vi "AO_master_Widefield_v0.vi"() -> ()   [LabVIEW 2018]
panel:
  in  "TurnOFFCooler":bool=TRUE caption="PD Correction"
  out "Return from GetStatus":u32
  in  "488 shutter":refnum<k7>(container)
  in  "Current Z as Center":bool=TRUE caption="PD Correction"
  in  "Z Step Num":i32=7
  in  "Z Step Size (um)":dbl=0.2
  in  "Spool":bool=TRUE caption="Cameras Live Display"
  in  "Acquire":bool
  in  "VISA Stage":refnum<visa-resource-name>="COM5"
  in  "Stage Options":bool
  in  "Auto Scale":bool=TRUE caption="PD Correction"
  out "Get EMCCD Gain":i32=1
  out "Return from SetSpool":i32=1
  out "Running Status":T1(ring) caption="Camera FOV"
  out "Return from Start Acquisition":u32
  out "Return from GetAcquiredData":u32
  in  "Folder Name":string="test"
  in  "File Type":enum16{"TIFF", "Sif"}(ring)
  out "Return from CheckProcess":u32
  out "Get Kinetic Time":sgl format="%.4f"
  out "Get Accum Time":sgl format="%.4f"
  out "Get Kinetic Num":i32=1
  out "Get Accum Num":i32=1
  in  "Abort":bool
  out "FOV Y Pixels":i32
  out "FOV X Pixels":i32
  in  "Snap":bool
  in  "Exit":bool
  out "EMCCD Status":bool
  in  "Stop LIVE":bool
  in  "Start LIVE":bool
  out "error out":errorcluster
  out "Return from CheckTimings":u32
  out "Get Exposure Time":sgl format="%.4f"
  in  "error in (no error)":errorcluster
  in  "Intensity Min":dbl=200.0 min=1.0
  in  "Intensity Max":dbl=10000.0 min=1.0
  in  "Shutdown EMCCD when exit":bool=TRUE caption="PD Correction"
  in  "Update FOV":bool
  in  "Update AcqSetting":bool
  in  "Exposure time (s)":dbl=0.02
  in  "Main Path":path=path "D:/Data"
  in  "File Name":string="test"
  in  "Kinetic Num":u32=1
  in  "Accum Num":u32=1
  in  "Initialize EMCCD":bool=TRUE caption="PD Correction"
  in  "CoolToTargetTemp":bool=TRUE caption="PD Correction"
  out "Intensity Graph":i32[][](graph)
  out "Current Temp":i32
  out "Detector Y Pixels":i32
  out "Detector X Pixels":i32
  in  "Aquisition Mode":T2(ring)=enum."Single Scan" caption="Camera FOV"
  in  "Trigger Mode":enum16{"Internal", "External"}(ring) caption="Camera FOV"
  in  "Gain Value":sgl=20.0 format="%.2f"
  in  "Yend":i32=1002
  in  "Xend":i32=1004
  in  "Ystart":i32=2
  in  "Xstart":i32=2
  in  "Ybin":i32=1
  in  "Xbin":i32=1
  in  "Camera FOV":T3(ring)=enum."Full FOV"
  in  "Gain On":bool=TRUE caption="Cameras Live Display"
  in  "Set Temp":i32=-60
  # "To do:\n1. make Kinetic work\n2. Gain setting\n3. live stage operation"
  # "It takes some time to cool down the camera before it shutdowns"
  # "C"
  # "Z move by relative position"
  # "Acquisition Settings"
  # "Status"
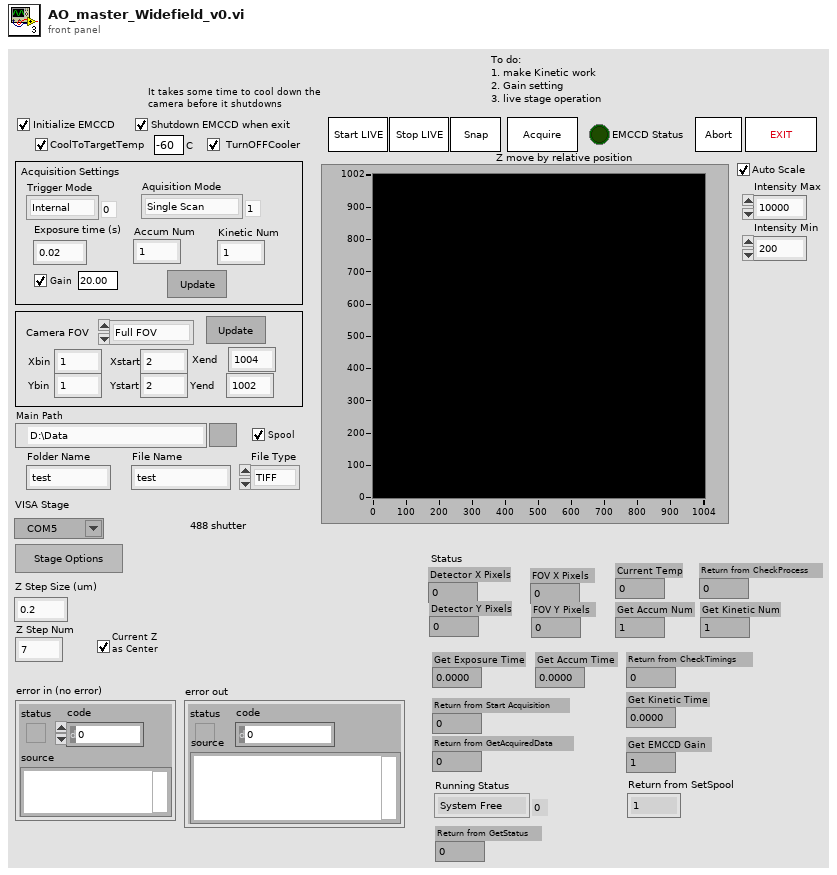
[diagram p1: front panel]
types:
  T1 = enum16{"System Free", "Live Preview", "Snap", " Acquisition", ""}
  T2 = enum16{"None", "Single Scan", "Accumulate", "Kinetics", "Fast Kinetics", "Run till abort"}
  T3 = enum16{"Custom FOV", "Full FOV", "FOV: 768x768", "FOV: 512x512", "FOV: 320x320", "FOV: 256x256", ""}
  T4 = typedef "Error Code Enum typedef.ctl" = enum32{"N/A (0)", "DRV_ERROR_CODES", "DRV_SUCCESS", "DRV_VXDNOTINSTALLED", "DRV_ERROR_SCAN", "DRV_ERROR_CHECK_SUM", "DRV_ERROR_FILELOAD", "DRV_UNKNOWN_FUNC", "DRV_ERROR_VXD_INIT", "DRV_ERROR_ADDRESS", "DRV_ERROR_PAGELOCK", "DRV_ERROR_PAGEUNLOCK", "DRV_ERROR_BOARDTEST", "DRV_ERROR_ACK", "DRV_ERROR_UP_FIFO", "DRV_ERROR_PATTERN", "N/A (16)", "DRV_ACQUISITION_ERRORS", "DRV_ACQ_BUFFER", "DRV_ACQ_DOWNFIFO_FULL", "DRV_PROC_UNKONWN_INSTRUCTION", "DRV_ILLEGAL_OP_CODE", "DRV_KINETIC_TIME_NOT_MET", "DRV_ACCUM_TIME_NOT_MET", "DRV_NO_NEW_DATA", "N/A (25)", "DRV_SPOOLERROR", "N/A (27)", "N/A (28)", "N/A (29)", "N/A (30)", "N/A (31)", "N/A (32)", "DRV_TEMPERATURE_CODES", "DRV_TEMPERATURE_OFF", "DRV_TEMPERATURE_NOT_STABILIZED", "DRV_TEMPERATURE_STABILIZED", "DRV_TEMPERATURE_NOT_REACHED", "DRV_TEMPERATURE_OUT_RANGE", "DRV_TEMPERATURE_NOT_SUPPORTED", "DRV_TEMPERATURE_DRIFT", "N/A (41)", "N/A (42)", "N/A (43)", "N/A (44)", "N/A (45)", "N/A (46)", "N/A (47)", "N/A (48)", "DRV_GENERAL_ERRORS", "DRV_INVALID_AUX", "DRV_COF_NOTLOADED", "DRV_FPGAPROG", "DRV_FLEXERROR", "DRV_GPIBERROR", "N/A (55)", "N/A (56)", "N/A (57)", "N/A (58)", "N/A (59)", "N/A (60)", "N/A (61)", "N/A (62)", "N/A (63)", "DRV_DATATYPE", "DRV_DRIVER_ERRORS", "DRV_P1INVALID", "DRV_P2INVALID", "DRV_P3INVALID", "DRV_P4INVALID", "DRV_INIERROR", "DRV_COFERROR", "DRV_ACQUIRING", "DRV_IDLE", "DRV_TEMPCYCLE", "DRV_NOT_INITIALIZED", "DRV_P5INVALID", "DRV_P6INVALID", "DRV_INVALID_MODE", "DRV_INVALID_FILTER", "DRV_I2CERRORS", "DRV_I2CDEVNOTFOUND", "DRV_I2CTIMEOUT", "DRV_P7INVALID", "N/A (84)", "N/A (85)", "N/A (86)", "N/A (87)", "N/A (88)", "N/A (89)", "DRV_IOCERROR", "DRV_VRMVERSIONERROR"}
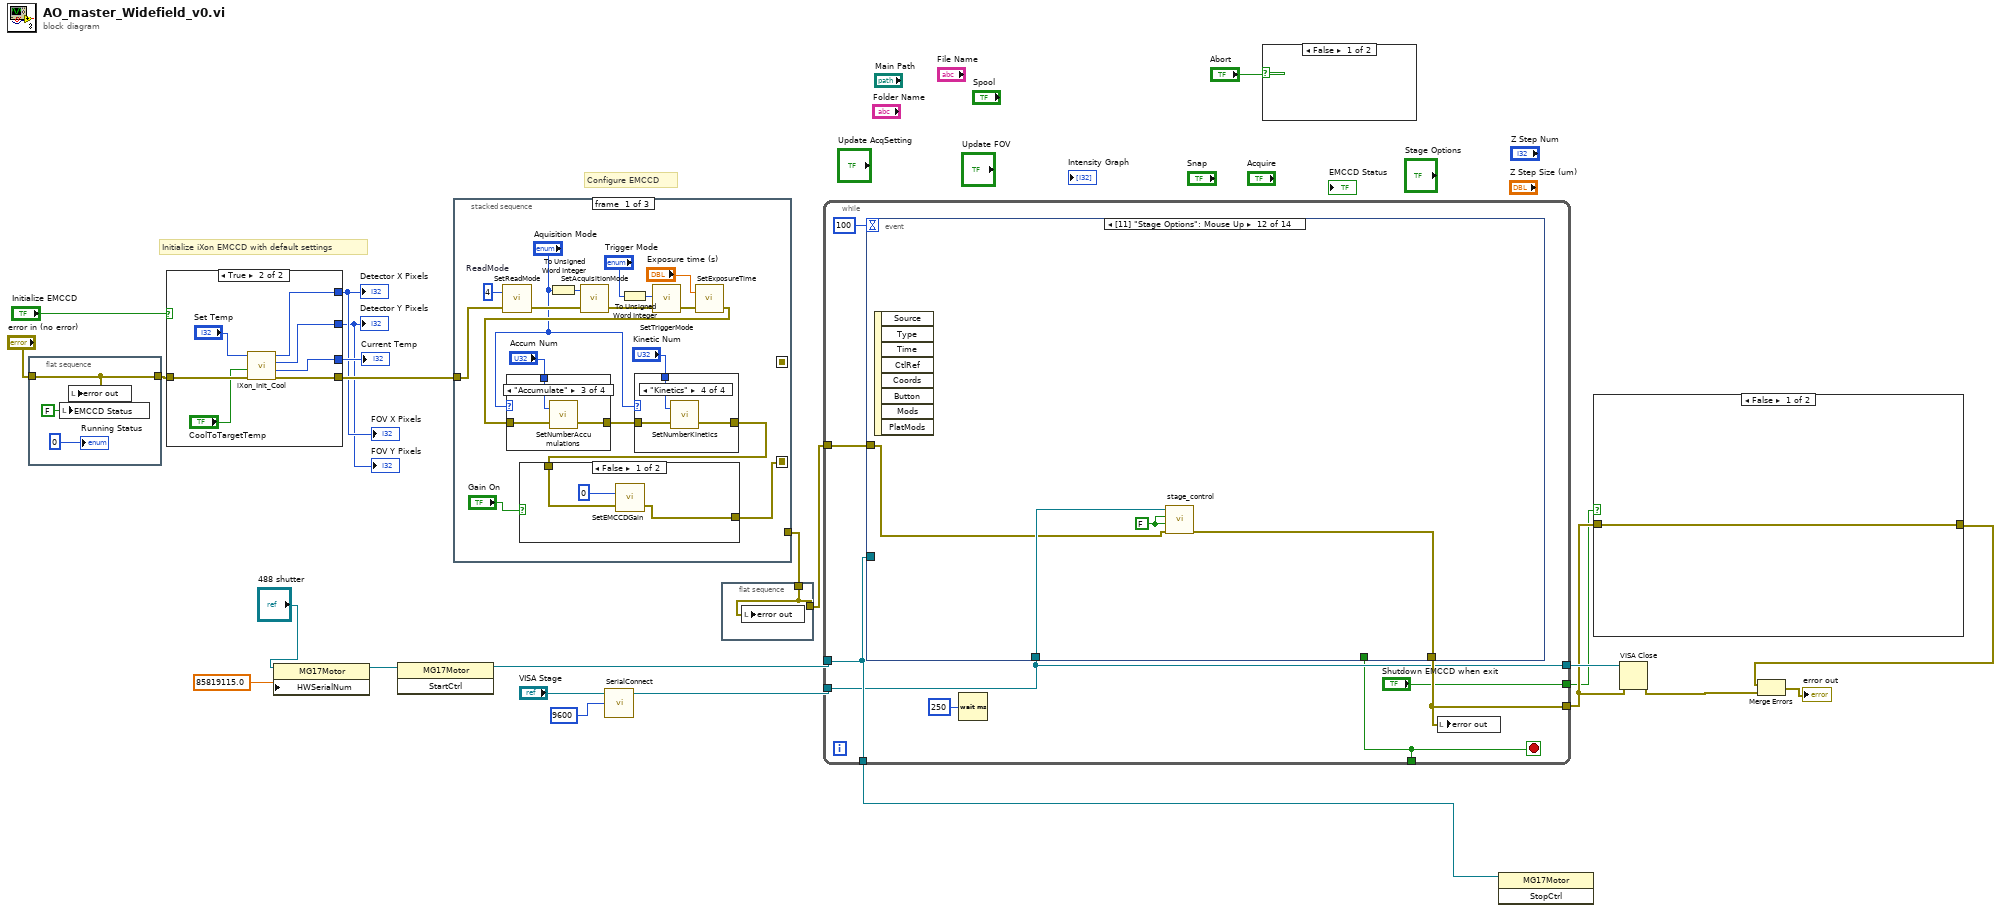
[diagram p0: block diagram]
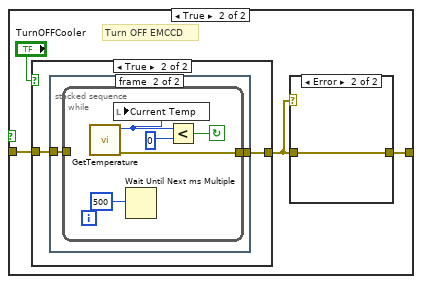
[diagram p2: hidden frame]
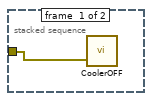
[diagram p4: hidden frame]
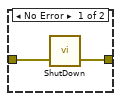
[diagram p5: hidden frame]
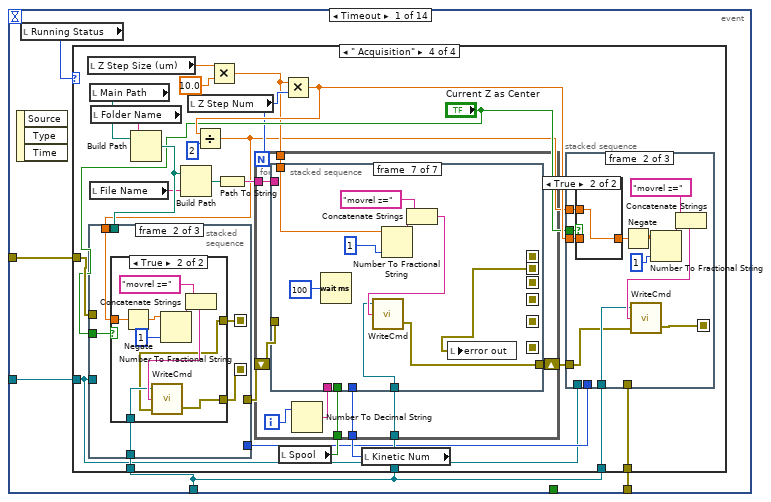
[diagram p7: hidden frame]
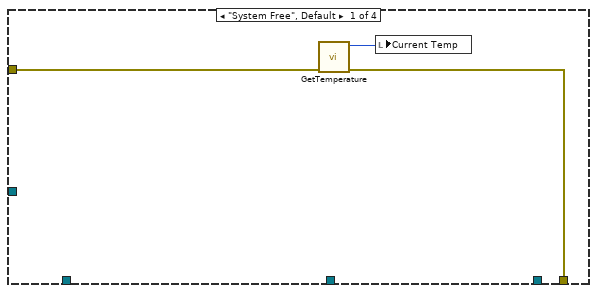
[diagram p8: hidden frame]
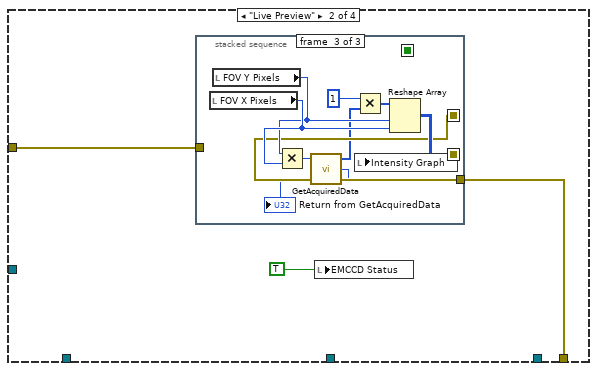
[diagram p9: hidden frame]
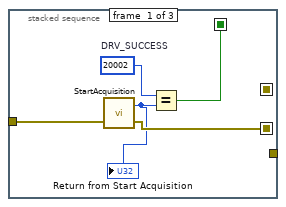
[diagram p10: hidden frame]
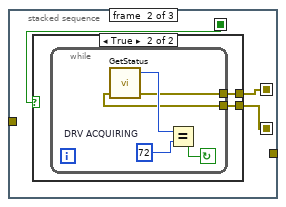
[diagram p11: hidden frame]
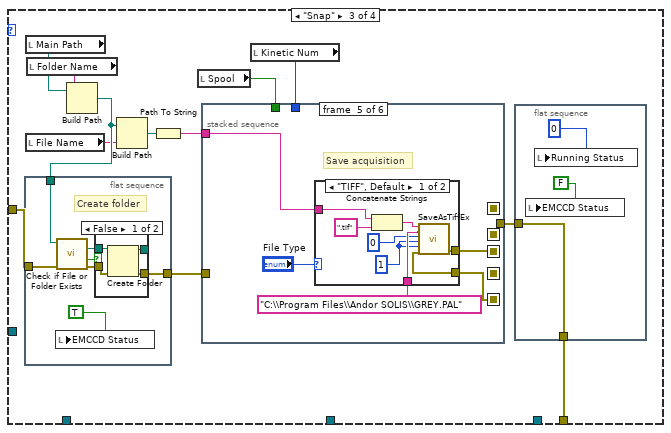
[diagram p13: hidden frame]
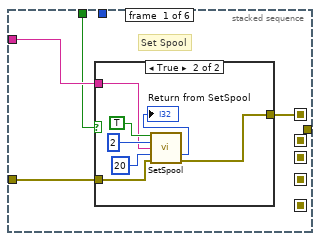
[diagram p14: hidden frame]
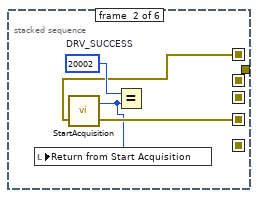
[diagram p16: hidden frame]
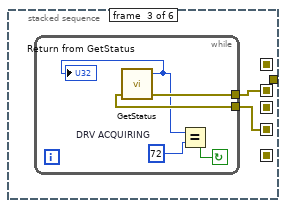
[diagram p17: hidden frame]
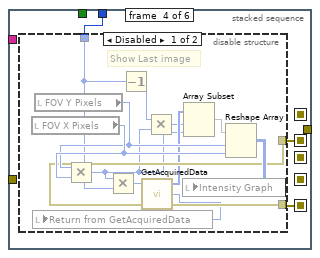
[diagram p18: hidden frame]
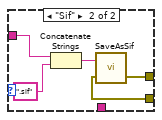
[diagram p20: hidden frame]
diagram:
  # "Configure EMCCD"
  # "Initialize iXon EMCCD with default settings"
  n1 = flat-sequence {
    tunnel: "error in (no error)" -> [w27]
    tunnel: [w27] -> w18
    frame #0 {
      n2 = local write "EMCCD Status"(FALSE) -> ()
      n3 = local write "error out"(w27) -> ()
      "Running Status" <- u16 0
    }
  }
  n4 = case shown="True" "Initialize EMCCD" {
    tunnel: w18 -> [w32 w39]
    tunnel: [w30 w37] -> w21
    tunnel: [w29 w36] -> w20
    tunnel: [w33 w35] -> w23
    tunnel: [w28 w34] -> w22
    frame False {
      n5 = call <userlib>:"GetDetector.vi"("error in (no error)"=w32) -> ("error out"=w31:errorcluster, "ypixels"=w29:i32, "xpixels"=w30:i32)  [unwired: 3 in, 1 out]
      n6 = call <userlib>:"GetTemperature.vi"("error in (no error)"=w31) -> ("error out"=w28:errorcluster, "temperature"=w33:i32)  [unwired: 3 in, 2 out]
    }
    frame True {
      n7 = call "iXon_Init_Cool.vi"("error in (no error)"=w39, "CoolToTargetTemp"="CoolToTargetTemp", "Set Temp"="Set Temp") -> ("error out"=w34:errorcluster, "Current Temp"=w35:i32, "Detector Y Pixels"=w36:i32, "Detector X Pixels"=w37:i32)  [unwired: 5 in]
    }
  }
  "Detector X Pixels" <- w21
  "Detector Y Pixels" <- w20
  "Current Temp" <- w23
  "FOV X Pixels" <- w21
  "FOV Y Pixels" <- w20
  n8 = property class="MG17Motor"(reference="488 shutter", "HWSerialNum"=85819115.0) -> (reference out=w10:refnum<k7>)  [unwired: 1 in, 1 out]
  n9 = invoke class="MG17Motor" method="StartCtrl"(reference=w10) -> (reference out=w7:refnum<k7>)  [unwired: 2 in, 2 out]
  n10 = stacked-sequence {
    seq-local: [w41 _ _] -> [_ w85 _]
    seq-local: [_ w84 _] -> [_ _ w183]
    tunnel: w22 -> [w55 _ _]
    tunnel: [_ _ w175] -> w17
    frame #0 {
      w56 = u16 4  # ReadMode
      n11 = call <userlib>:"SetReadMode.vi"("error in (no error)"=w55, "mode"=w56) -> ("error out"=w53:errorcluster)  [unwired: 1 out]
      n12 = To Unsigned Word Integer(number="Aquisition Mode") -> (unsigned 16bit integer=w57:u16)
      n13 = call <userlib>:"SetAcquisitionMode.vi"("error in (no error)"=w53, "mode"=w57) -> ("error out"=w52:errorcluster)  [unwired: 1 out]
      n14 = To Unsigned Word Integer(number="Trigger Mode") -> (unsigned 16bit integer=w51:u16)
      n15 = call <userlib>:"SetTriggerMode.vi"("error in (no error)"=w52, "mode"=w51) -> ("error out"=w50:errorcluster)  [unwired: 1 out]
      n16 = call <userlib>:"SetExposureTime.vi"("error in (no error)"=w50, "time"="Exposure time (s)") -> ("error out"=w47:errorcluster)  [unwired: 1 out]
      n17 = case shown="\"Accumulate\"" "Aquisition Mode" {
        tunnel: "Accum Num" -> [_ _ w76 w79]
        tunnel: w47 -> [w72 w73 w75 w78]
        tunnel: [w72 w73 w74 w77] -> w46
        frame "None", Default {
        }
        frame "Single Scan" {
        }
        frame "Accumulate" {
          n18 = call <userlib>:"SetNumberAccumulations.vi"("error in (no error)"=w75, "number"=w76) -> ("error out"=w74:errorcluster)  [unwired: 1 out]
        }
        frame "Kinetics" {
          n19 = call <userlib>:"SetNumberAccumulations.vi"("error in (no error)"=w78, "number"=w79) -> ("error out"=w77:errorcluster)  [unwired: 1 out]
        }
      }
      n20 = case shown="\"Kinetics\"" "Aquisition Mode" {
        tunnel: w46 -> [w66 w67 w68 w71]
        tunnel: [w66 w67 w68 w70] -> w42
        tunnel: "Kinetic Num" -> [_ _ _ w69]
        frame "None", Default {
        }
        frame "Single Scan" {
        }
        frame "Accumulate" {
        }
        frame "Kinetics" {
          n21 = call <userlib>:"SetNumberKinetics.vi"("error in (no error)"=w71, "number"=w69) -> ("error out"=w70:errorcluster)  [unwired: 1 out]
        }
      }
      n22 = case shown="False" "Gain On" {
        tunnel: w42 -> [w59 w65]
        tunnel: [w58 w62] -> w41
        frame False {
          n23 = call <userlib>:"SetEMCCDGain.vi"("error in (no error)"=w59, "gain"=0) -> ("error out"=w58:errorcluster)  [unwired: 1 out]
        }
        frame True {
          # "0-255"
          n24 = call <userlib>:"SetEMGainMode.vi"("error in (no error)"=w65, "mode"=0) -> ("error out"=w63:errorcluster)  [unwired: 1 out]
          n25 = call <userlib>:"SetEMCCDGain.vi"("error in (no error)"=w63, "gain"="Gain Value") -> ("error out"=w62:errorcluster)  [unwired: 1 out]
        }
      }
    }
    frame #1 {
      # "Set FOV"
      n26 = local read "Detector X Pixels"() -> (w83:i32)
      n27 = local read "Detector Y Pixels"() -> (w82:i32)
      n28 = case shown="\"Custom FOV\"" "Camera FOV" {
        tunnel: ["Xbin" w122 w138 w154 w170 w173] -> w91
        tunnel: ["Ybin" w122 w138 w154 w170 w173] -> w90
        tunnel: ["Xstart" w112 w128 w144 w160 w173] -> w89
        tunnel: ["Xend" w109 w125 w141 w157 w171] -> w88
        tunnel: ["Ystart" w111 w127 w143 w159 w173] -> w87
        tunnel: ["Yend" w108 w124 w140 w156 w172] -> w86
        tunnel: w83 -> [_ w121 w137 w153 w169 w171]
        tunnel: w82 -> [_ w120 w136 w152 w168 w172]
        tunnel: [w93 w107 w123 w139 w155 w172] -> w81
        tunnel: [w96 w107 w123 w139 w155 w171] -> w80
        frame "Custom FOV" {
          n29 = Subtract(x="Yend", y="Ystart") -> (x-y=w103:i32)
          n30 = Subtract(x="Xend", y="Xstart") -> (x-y=w106:i32)
          n31 = Increment(x=w103) -> (x+1=w100:i32)
          n32 = Increment(x=w106) -> (x+1=w99:i32)
          n33 = Divide(x=w100, y="Ybin") -> (x/y=w94:dbl)
          n34 = Divide(x=w99, y="Xbin") -> (x/y=w97:dbl)
          n35 = To Long Integer(number=w94) -> (32bit integer=w93:i32)
          n36 = To Long Integer(number=w97) -> (32bit integer=w96:i32)
        }
        frame "FOV: 768x768" {
          w107 = 768
          w117 = 2.0
          w122 = 1
          n37 = Subtract(x=w121, y=w107) -> (x-y=w119:i32)
          n38 = Subtract(x=w120, y=w107) -> (x-y=w118:i32)
          n39 = Divide(x=w118, y=w117) -> (x/y=w115:dbl)
          n40 = Divide(x=w119, y=w117) -> (x/y=w116:dbl)
          n41 = Decrement(x=w107) -> (x-1=w110:i32)
          n42 = Round To Nearest(number=w116) -> (nearest integer value=w114:dbl)
          n43 = Round To Nearest(number=w115) -> (nearest integer value=w113:dbl)
          n44 = To Long Integer(number=w114) -> (32bit integer=w112:i32)
          n45 = To Long Integer(number=w113) -> (32bit integer=w111:i32)
          n46 = Add(x=w110, y=w112) -> (x+y=w109:i32)
          n47 = Add(x=w110, y=w111) -> (x+y=w108:i32)
        }
        frame "FOV: 512x512" {
          w123 = 512
          w133 = 2.0
          w138 = 1
          n48 = Subtract(x=w137, y=w123) -> (x-y=w135:i32)
          n49 = Subtract(x=w136, y=w123) -> (x-y=w134:i32)
          n50 = Divide(x=w134, y=w133) -> (x/y=w131:dbl)
          n51 = Divide(x=w135, y=w133) -> (x/y=w132:dbl)
          n52 = Decrement(x=w123) -> (x-1=w126:i32)
          n53 = Round To Nearest(number=w132) -> (nearest integer value=w130:dbl)
          n54 = Round To Nearest(number=w131) -> (nearest integer value=w129:dbl)
          n55 = To Long Integer(number=w130) -> (32bit integer=w128:i32)
          n56 = To Long Integer(number=w129) -> (32bit integer=w127:i32)
          n57 = Add(x=w126, y=w128) -> (x+y=w125:i32)
          n58 = Add(x=w126, y=w127) -> (x+y=w124:i32)
        }
        frame "FOV: 320x320" {
          w139 = 320
          w149 = 2.0
          w154 = 1
          n59 = Subtract(x=w153, y=w139) -> (x-y=w151:i32)
          n60 = Subtract(x=w152, y=w139) -> (x-y=w150:i32)
          n61 = Divide(x=w150, y=w149) -> (x/y=w147:dbl)
          n62 = Divide(x=w151, y=w149) -> (x/y=w148:dbl)
          n63 = Decrement(x=w139) -> (x-1=w142:i32)
          n64 = Round To Nearest(number=w148) -> (nearest integer value=w146:dbl)
          n65 = Round To Nearest(number=w147) -> (nearest integer value=w145:dbl)
          n66 = To Long Integer(number=w146) -> (32bit integer=w144:i32)
          n67 = To Long Integer(number=w145) -> (32bit integer=w143:i32)
          n68 = Add(x=w142, y=w144) -> (x+y=w141:i32)
          n69 = Add(x=w142, y=w143) -> (x+y=w140:i32)
        }
        frame "FOV: 256x256" {
          w155 = 256
          w165 = 2.0
          w170 = 1
          n70 = Subtract(x=w169, y=w155) -> (x-y=w167:i32)
          n71 = Subtract(x=w168, y=w155) -> (x-y=w166:i32)
          n72 = Divide(x=w166, y=w165) -> (x/y=w163:dbl)
          n73 = Divide(x=w167, y=w165) -> (x/y=w164:dbl)
          n74 = Decrement(x=w155) -> (x-1=w158:i32)
          n75 = Round To Nearest(number=w164) -> (nearest integer value=w162:dbl)
          n76 = Round To Nearest(number=w163) -> (nearest integer value=w161:dbl)
          n77 = To Long Integer(number=w162) -> (32bit integer=w160:i32)
          n78 = To Long Integer(number=w161) -> (32bit integer=w159:i32)
          n79 = Add(x=w158, y=w160) -> (x+y=w157:i32)
          n80 = Add(x=w158, y=w159) -> (x+y=w156:i32)
        }
        frame "Full FOV", Default {
          w173 = 1
        }
      }
      n81 = local write "FOV X Pixels"(w80) -> ()
      n82 = local write "FOV Y Pixels"(w81) -> ()
      n83 = call <userlib>:"SetImage.vi"("hbin"=w91, "vbin"=w90, "hstart"=w89, "hend"=w88, "vstart"=w87, "vend"=w86, "error in (no error)"=w85) -> ("error out"=w84:errorcluster)  [unwired: 19 in, 1 out]
    }
    frame #2 {
      n84 = call <userlib>:"GetAcquisitionTimings.vi"("error in (no error)"=w183) -> ("exposure"=→"Get Exposure Time":sgl, "accumulate"=→"Get Accum Time":sgl, "kinetic"=→"Get Kinetic Time":sgl, "DLL error code"=→"Return from CheckTimings":u32, "error out"=w182:errorcluster)  [unwired: 10 in]
      n85 = call <userlib>:"GetAcquisitionProgress.vi"("error in (no error)"=w182) -> ("error out"=w176:errorcluster, "DLL error code"=→"Return from CheckProcess":u32, "series"=→"Get Kinetic Num":i32, "accum"=→"Get Accum Num":i32)  [unwired: 3 in]
      n86 = call <userlib>:"GetEMCCDGain.vi"("error in (no error)"=w176) -> ("error out"=w175:errorcluster, "gain"=→"Get EMCCD Gain":u32)  [unwired: 2 in, 1 out]
    }
  }
  n87 = call "SerialConnect.vi"("baud rate (9600)"=9600, "VISA resource name"="VISA Stage") -> ("VISA out"=w4:refnum<visa-resource-name>)  [unwired: 1 in, 2 out]
  n88 = flat-sequence {
    tunnel: w17 -> [w186]
    tunnel: [w186] -> w5
    frame #0 {
      n89 = local write "error out"(w186) -> ()
    }
  }
  n90 = while {
    tunnel: w5 -> [w188]
    tunnel: [w193] -> w3
    tunnel: ["Shutdown EMCCD when exit"] -> w1
    tunnel: w4 -> [w189]
    tunnel: [w189] -> w13
    tunnel: w7 -> [w190]
    tunnel: [w190] -> w6
    tunnel: [w187] -> _
    stop <- w187 stop-if-true
    n91 = event shown="[11] \"Stage Options\": Mouse Up" {
      selector: _ -> [_ _ _ _ _ _ _ _ _ _ _ _ _ _]
      dyn-events: _ -> [_ _ _ _ _ _ _ _ _ _ _ _ _ _]
      timeout: 100 -> [_ _ _ _ _ _ _ _ _ _ _ _ _ _]
      tunnel: w188 -> [w197 w510 w548 w643 w652 w661 w663 w666 w669 w671 w673 w675 w678 w681]
      tunnel: [w198 w508 w545 w642 w650 w661 w663 w665 w669 w671 w673 w674 w678 w681] -> w193
      tunnel: [_ _ _ _ _ _ _ _ _ _ _ _ TRUE ("Exit") TRUE ("Exit")] -> w187
      tunnel: w189 -> [w196 _ _ _ _ _ _ _ _ _ _ w676 _ _]
      tunnel: w190 -> [w195 _ _ _ _ _ _ _ _ _ _ _ _ _]
      event Timeout {
        n92 = event-data() -> ()  [unwired: 1 in, 3 out]
        n93 = local read "Running Status"() -> (w199:T1)
        n94 = case shown="\" Acquisition\"" w199 {
          tunnel: [w200 w205 w241 w351] -> w198
          tunnel: w197 -> [w201 w204 w240 w350]
          tunnel: w196 -> [_ _ _ w338]
          tunnel: w196 -> [_ _ _ w336]
          tunnel: w196 -> [_ _ _ w335]
          tunnel: w195 -> [_ _ _ w330]
          frame "System Free", Default {
            n95 = call <userlib>:"GetTemperature.vi"("error in (no error)"=w201) -> ("error out"=w200:errorcluster, "temperature"=w202:i32)  [unwired: 3 in, 2 out]
            n96 = local write "Current Temp"(w202) -> ()
          }
          frame "Live Preview" {
            n97 = stacked-sequence {
              seq-local: [w208 _ _] -> [_ w213 _]
              seq-local: [_ w212 _] -> [_ _ w227]
              seq-local: [w207 _ _] -> [_ w211 _]
              tunnel: w204 -> [w209 _ _]
              tunnel: [_ _ w226] -> w205
              frame #0 {
                w210 = 20002  # DRV_SUCCESS
                n98 = call <userlib>:"StartAcquisition.vi"("error in (no error)"=w209) -> ("error out"=w208:errorcluster, "DLL error code"=w206:u32)  [unwired: 1 in]
                "Return from Start Acquisition" <- w206
                n99 = Equal?(x=w210, y=w206) -> (x = y?=w207:bool)
              }
              frame #1 {
                n100 = case shown="True" w211 {
                  tunnel: w213 -> [w214 w216]
                  tunnel: [w214 w215] -> w212
                  frame False {
                  }
                  frame True {
                    n101 = while {
                      tunnel: w216 -> [w218]
                      tunnel: [w217] -> w215
                      stop <- w219 continue-if-true
                      w221 = u16 72  # DRV ACQUIRING
                      n102 = call <userlib>:"GetStatus.vi"("error in (no error)"=w218) -> ("error out"=w217:errorcluster, "status"=w220:T4)  [unwired: 2 in, 1 out]
                      n103 = Equal?(x=w220, y=w221) -> (x = y?=w219:bool)
                    }
                  }
                }
              }
              frame #2 {
                n104 = local read "FOV X Pixels"() -> (w230:i32)
                n105 = local read "FOV Y Pixels"() -> (w229:i32)
                n106 = Multiply(x=w229, y=w230) -> (x*y=w231:i32)
                n107 = call <userlib>:"GetAcquiredData.vi"("error in (no error)"=w227, "size"=w231) -> ("error out"=w226:errorcluster, "DLL error code"=→"Return from GetAcquiredData":u32, "array"=w222:i32[])  [unwired: 1 in]
                n108 = Multiply(x=1, y=w222) -> (x*y=w223:i32[])
                n109 = Reshape Array(w223, w229, w230) -> (w228:i32[][])
                n110 = local write "Intensity Graph"(w228) -> ()
              }
            }
            n111 = local write "EMCCD Status"(TRUE) -> ()
          }
          frame "Snap" {
            n112 = flat-sequence {
              tunnel: [w315] -> w243
              tunnel: w240 -> [w317]
              tunnel: w242 -> [w318]
              frame #0 {
                # "Create folder"
                n113 = local write "EMCCD Status"(TRUE) -> ()
                n114 = call <vilib>:"Check if File or Folder Exists.vi"("error in (no error)"=w317, "path"=w318) -> ("error out"=w316:errorcluster, "file or folder exists?"=w320:bool, "dup path"=w319:path)  [unwired: 7 in]
                n115 = case shown="False" w320 {
                  tunnel: w319 -> [w325 w327]
                  tunnel: [w324 w327] -> _
                  tunnel: w316 -> [w323 w326]
                  tunnel: [w322 w326] -> w315
                  frame False {
                    n116 = Create Folder(path (use dialog)=w325, error in=w323) -> (created path=w324:path, error out=w322:errorcluster)  [unwired: 1 in, 1 out]
                  }
                  frame True {
                  }
                }
              }
            }
            n117 = local read "Main Path"() -> (w234:path)
            n118 = local read "File Name"() -> (w232:string)
            n119 = local read "Folder Name"() -> (w233:string)
            n120 = Build Path(base path=w234, name or relative path=w233) -> (appended path=w242:path)
            n121 = Build Path(base path=w242, name or relative path=w232) -> (appended path=w239:path)
            n122 = Path To String(path=w239) -> (string=w238:string)
            n123 = local read "Spool"() -> (w235:bool)
            n124 = local read "Kinetic Num"() -> (w237:u32)
            n125 = stacked-sequence {
              seq-local: [_ w258 _ _ _ _] -> [_ _ w261 _ _ _]
              seq-local: [_ _ w260 _ _ _] -> [_ _ _ w269 _ _]
              seq-local: [_ _ _ w268 _ _] -> [_ _ _ _ w286 _]
              seq-local: [w245 _ _ _ _ _] -> [_ w257 _ _ _ _]
              seq-local: [_ _ _ _ w284 _] -> [_ _ _ _ _ w305]
              tunnel: w243 -> [w246 _ _ _ _ _]
              tunnel: w238 -> [w247 _ _ _ w285 w303]
              tunnel: w237 -> [_ _ _ w267 _ w306]
              tunnel: w235 -> [w244 _ _ _ _ w302]
              tunnel: [_ _ _ _ _ w304] -> w236
              frame #0 {
                # "Set Spool"
                n126 = case shown="True" w244 {
                  tunnel: w247 -> [_ w252]
                  tunnel: w246 -> [w248 w251]
                  tunnel: [w248 w249] -> w245
                  frame False {
                  }
                  frame True {
                    n127 = call <userlib>:"SetSpool.vi"("active"=TRUE, "method"=2, "name"=w252, "framebuffersize (10)"=20, "error in (no error)"=w251) -> ("DLL error code"=→"Return from SetSpool":u32, "error out"=w249:errorcluster)  [unwired: 9 in]
                  }
                }
              }
              frame #1 {
                w259 = 20002  # DRV_SUCCESS
                n128 = call <userlib>:"StartAcquisition.vi"("error in (no error)"=w257) -> ("error out"=w258:errorcluster, "DLL error code"=w256:u32)  [unwired: 1 in]
                n129 = local write "Return from Start Acquisition"(w256) -> ()
                n130 = Equal?(x=w259, y=w256) -> ()  [unwired: 1 out]
              }
              frame #2 {
                n131 = while {
                  tunnel: w261 -> [w264]
                  tunnel: [w263] -> w260
                  stop <- w265 continue-if-true
                  w266 = u16 72  # DRV ACQUIRING
                  n132 = call <userlib>:"GetStatus.vi"("error in (no error)"=w264) -> ("error out"=w263:errorcluster, "status"=w262:T4)  [unwired: 2 in, 1 out]
                  "Return from GetStatus" <- w262
                  n133 = Equal?(x=w262, y=w266) -> (x = y?=w265:bool)
                }
              }
              frame #3 {
                n134 = disable-structure shown="Disabled" {
                  disable-tunnel: w269 -> [w279 w283]
                  disable-tunnel: [w274 w283] -> w268
                  disable-tunnel: w267 -> [w271 _]
                  frame Disabled {
                    # "Show Last image"
                    n135 = local read "FOV X Pixels"() -> (w282:i32)
                    n136 = local read "FOV Y Pixels"() -> (w281:i32)
                    n137 = Multiply(x=w281, y=w282) -> (x*y=w272:i32)
                    n138 = Multiply(x=w272, y=w271) -> (x*y=w273:u32)
                    n139 = Decrement(x=w271) -> (x-1=w275:u32)
                    n140 = call <userlib>:"GetAcquiredData.vi"("error in (no error)"=w279, "size"=w273) -> ("error out"=w274:errorcluster, "DLL error code"=w270:u32, "array"=w278:i32[])  [unwired: 1 in]
                    n141 = local write "Return from GetAcquiredData"(w270) -> ()
                    n142 = Multiply(x=w275, y=w272) -> (x*y=w276:u32)
                    n143 = Array Subset(array=w278, index=w276, length=w272) -> (w277:i32[])
                    n144 = Reshape Array(w277, w281, w282) -> (w280:i32[][])
                    n145 = local write "Intensity Graph"(w280) -> ()
                  }
                  frame Enabled {
                  }
                }
              }
              frame #4 {
                # "Save acquisition"
                n146 = case shown="\"TIFF\", Default" "File Type" {
                  tunnel: "C:\\Program Files\\Andor SOLIS\\GREY.PAL" -> [w292 _]
                  tunnel: w285 -> [w295 w301]
                  tunnel: w286 -> [w293 w298]
                  tunnel: [w294 w297] -> w284
                  frame "TIFF", Default {
                    w289 = 1
                    n147 = Concatenate Strings(w295, ".tif") -> (w291:string)
                    n148 = call <userlib>:"SaveAsTiffEx.vi"("path"=w291, "palette"=w292, "position"=0, "type"=w289, "mode"=w289, "error in (no error)"=w293) -> ("error out"=w294:errorcluster)  [unwired: 12 in, 1 out]
                  }
                  frame "Sif" {
                    n149 = Concatenate Strings(w301, ".sif") -> (w299:string)
                    n150 = call <userlib>:"SaveAsSif.vi"("error in (no error)"=w298, "path"=w299) -> ("error out"=w297:errorcluster)  [unwired: 1 out]
                  }
                }
              }
              frame #5 {
                # "Clearn Spool Files"
                n151 = case shown="True" w302 {
                  tunnel: w306 -> [_ w311]
                  tunnel: w305 -> [w307 w310]
                  tunnel: [w307 w309] -> w304
                  tunnel: w303 -> [_ w308]
                  frame False {
                  }
                  frame True {
                    n152 = call "cleanSpool.vi"("error in (no error)"=w310, "Total Img Num"=w311, "strPath"=w308) -> ("error out"=w309:errorcluster)  [unwired: 8 in]
                  }
                }
              }
            }
            n153 = flat-sequence {
              tunnel: w236 -> [w313]
              tunnel: [w313] -> w241
              frame #0 {
                n154 = local write "EMCCD Status"(FALSE) -> ()
                n155 = local write "Running Status"(0) -> ()
              }
            }
          }
          frame " Acquisition" {
            n156 = local read "Z Step Size (um)"() -> (w342:dbl)
            n157 = local read "Main Path"() -> (w345:path)
            n158 = local read "File Name"() -> (w343:string)
            n159 = local read "Folder Name"() -> (w344:string)
            n160 = Build Path(base path=w345, name or relative path=w344) -> (appended path=w352:path)
            n161 = Build Path(base path=w352, name or relative path=w343) -> (appended path=w349:path)
            n162 = local read "Z Step Num"() -> (w332:i32)
            n163 = Multiply(x=w342, y=10.0) -> (x*y=w329:dbl)
            n164 = Path To String(path=w349) -> (string=w348:string)
            n165 = local read "Spool"() -> (w346:bool)
            n166 = Multiply(x=w329, y=w332) -> (x*y=w339:dbl)
            n167 = Divide(x=w339, y=2) -> (x/y=w328:dbl)
            n168 = stacked-sequence {
              seq-local: [w465 _ _] -> [_ w479 _]
              seq-local: [_ w478 _] -> [_ _ w497]
              tunnel: w350 -> [w467 _ _]
              tunnel: w352 -> [w468 _ _]
              tunnel: [_ _ w495] -> w337
              tunnel: w328 -> [_ w482 _]
              tunnel: w336 -> [_ w481 _]
              tunnel: "Current Z as Center" -> [_ w480 _]
              tunnel: w330 -> [_ _ w496]
              tunnel: [_ _ w494] -> w331
              frame #0 {
                # "Create folder"
                n169 = local write "EMCCD Status"(TRUE) -> ()
                n170 = call <vilib>:"Check if File or Folder Exists.vi"("error in (no error)"=w467, "path"=w468) -> ("error out"=w466:errorcluster, "file or folder exists?"=w470:bool, "dup path"=w469:path)  [unwired: 7 in]
                n171 = case shown="False" w470 {
                  tunnel: w469 -> [w475 w477]
                  tunnel: [w474 w477] -> _
                  tunnel: w466 -> [w473 w476]
                  tunnel: [w472 w476] -> w465
                  frame False {
                    n172 = Create Folder(path (use dialog)=w475, error in=w473) -> (created path=w474:path, error out=w472:errorcluster)  [unwired: 1 in, 1 out]
                  }
                  frame True {
                  }
                }
              }
              frame #1 {
                n173 = case shown="True" w480 {
                  tunnel: [w483 w488] -> w478
                  tunnel: w482 -> [_ w487]
                  tunnel: w481 -> [_ w486]
                  tunnel: w479 -> [w483 w485]
                  frame False {
                  }
                  frame True {
                    n174 = Negate(x=w487) -> (-x=w492:dbl)
                    n175 = Number To Fractional String(number=w492, precision (6)=1) -> (F-format string=w491:string)  [unwired: 2 in]
                    n176 = Concatenate Strings("movrel z=", w491) -> (w490:string)
                    n177 = call "WriteCmd.vi"("error IO"=w485, "Command"=w490, "VISA resource name"=w486) -> ("error"=w488:errorcluster)  [unwired: 1 out]
                  }
                }
              }
              frame #2 {
                # "Turn on laser"
                n178 = invoke class="MG17Motor" method="SC_Enable"(reference=w496, error in=w497, "lChanID"=0) -> (error out=w495:errorcluster, "lChanID"=w494:i32)  [unwired: 1 in, 2 out]
                n179 = Wait (ms)(milliseconds to wait=u32 1000) -> ()  [unwired: 1 out]
              }
            }
            n180 = local read "Kinetic Num"() -> (w347:u32)
            n181 = for {
              N: w332 -> [_]
              tunnel: w348 -> [w361]
              tunnel: w347 -> [w360]
              tunnel: w346 -> [w359]
              tunnel: w335 -> [w357]
              tunnel: w329 -> [w355]
              shift-right: [w356] -> w334
              shift-left: w337 -> [w358]
              i -> [w354]
              n182 = Number To Decimal String(number=w354) -> (decimal integer string=w353:string)  [unwired: 1 in]
              n183 = stacked-sequence {
                seq-local: [_ w376 _ _ _ _ _] -> [_ _ w380 _ _ _ _]
                seq-local: [_ _ w379 _ _ _ _] -> [_ _ _ w388 _ _ _]
                seq-local: [_ _ _ w387 _ _ _] -> [_ _ _ _ w408 _ _]
                seq-local: [w364 _ _ _ _ _ _] -> [_ w375 _ _ _ _ _]
                seq-local: [_ _ _ _ w407 _ _] -> [_ _ _ _ _ w429 _]
                seq-local: [_ _ _ _ _ w427 _] -> [_ _ _ _ _ _ w436]
                tunnel: w358 -> [w365 _ _ _ _ _ _]
                tunnel: w361 -> [w366 _ _ _ w404 w424 _]
                tunnel: w360 -> [_ _ _ w386 _ w430 _]
                tunnel: w359 -> [w363 _ _ _ _ w428 _]
                tunnel: w357 -> [_ _ _ _ _ _ w441]
                tunnel: [_ _ _ _ _ _ w440] -> w356
                tunnel: w355 -> [_ _ _ _ _ _ w439]
                tunnel: w353 -> [_ _ _ _ w402 w425 _]
                frame #0 {
                  # "Set Spool"
                  n184 = Wait (ms)(milliseconds to wait=u32 100) -> ()  [unwired: 1 out]
                  n185 = case shown="True" w363 {
                    tunnel: w366 -> [_ w371]
                    tunnel: w365 -> [w367 w370]
                    tunnel: [w367 w369] -> w364
                    frame False {
                    }
                    frame True {
                      n186 = call <userlib>:"SetSpool.vi"("active"=TRUE, "method"=2, "name"=w371, "framebuffersize (10)"=20, "error in (no error)"=w370) -> ("DLL error code"=w368:u32, "error out"=w369:errorcluster)  [unwired: 9 in]
                      n187 = local write "Return from SetSpool"(w368) -> ()
                    }
                  }
                }
                frame #1 {
                  w377 = 20002  # DRV_SUCCESS
                  n188 = call <userlib>:"StartAcquisition.vi"("error in (no error)"=w375) -> ("error out"=w376:errorcluster, "DLL error code"=w378:u32)  [unwired: 1 in]
                  n189 = Equal?(x=w377, y=w378) -> ()  [unwired: 1 out]
                }
                frame #2 {
                  n190 = while {
                    tunnel: w380 -> [w382]
                    tunnel: [w381] -> w379
                    stop <- w383 continue-if-true
                    w385 = u16 72  # DRV ACQUIRING
                    n191 = call <userlib>:"GetStatus.vi"("error in (no error)"=w382) -> ("error out"=w381:errorcluster, "status"=w384:T4)  [unwired: 2 in, 1 out]
                    n192 = Equal?(x=w384, y=w385) -> (x = y?=w383:bool)
                  }
                }
                frame #3 {
                  n193 = disable-structure shown="Enabled" {
                    disable-tunnel: w388 -> [w397 w401]
                    disable-tunnel: [w392 w401] -> w387
                    disable-tunnel: w386 -> [w389 _]
                    frame Disabled {
                      # "Show Last image"
                      n194 = local read "FOV X Pixels"() -> (w400:i32)
                      n195 = local read "FOV Y Pixels"() -> (w399:i32)
                      n196 = Multiply(x=w399, y=w400) -> (x*y=w390:i32)
                      n197 = Multiply(x=w390, y=w389) -> (x*y=w391:u32)
                      n198 = Decrement(x=w389) -> (x-1=w393:u32)
                      n199 = call <userlib>:"GetAcquiredData.vi"("error in (no error)"=w397, "size"=w391) -> ("error out"=w392:errorcluster, "array"=w396:i32[])  [unwired: 1 in, 1 out]
                      n200 = Multiply(x=w393, y=w390) -> (x*y=w394:u32)
                      n201 = Array Subset(array=w396, index=w394, length=w390) -> (w395:i32[])
                      n202 = Reshape Array(w395, w399, w400) -> (w398:i32[][])
                      n203 = local write "Intensity Graph"(w398) -> ()
                    }
                    frame Enabled {
                    }
                  }
                }
                frame #4 {
                  # "Save acquisition"
                  n204 = local read "File Type"() -> (w406:enum16{"TIFF", "Sif"})
                  n205 = Concatenate Strings(w404, "_", w402) -> (w405:string)
                  n206 = case shown="\"TIFF\", Default" w406 {
                    tunnel: "C:\\Program Files\\Andor SOLIS\\GREY.PAL" -> [w413 _]
                    tunnel: w405 -> [w416 w422]
                    tunnel: w408 -> [w414 w419]
                    tunnel: [w415 w418] -> w407
                    frame "TIFF", Default {
                      w410 = 1
                      n207 = Concatenate Strings(w416, ".tif") -> (w412:string)
                      n208 = call <userlib>:"SaveAsTiffEx.vi"("path"=w412, "palette"=w413, "position"=0, "type"=w410, "mode"=w410, "error in (no error)"=w414) -> ("error out"=w415:errorcluster)  [unwired: 12 in, 1 out]
                    }
                    frame "Sif" {
                      n209 = Concatenate Strings(w422, ".sif") -> (w420:string)
                      n210 = call <userlib>:"SaveAsSif.vi"("error in (no error)"=w419, "path"=w420) -> ("error out"=w418:errorcluster)  [unwired: 1 out]
                    }
                  }
                }
                frame #5 {
                  # "Clearn Spool Files"
                  n211 = Concatenate Strings(w424, "_", w425) -> (w426:string)
                  n212 = case shown="True" w428 {
                    tunnel: w430 -> [_ w435]
                    tunnel: w429 -> [w431 w434]
                    tunnel: [w431 w433] -> w427
                    tunnel: w426 -> [_ w432]
                    frame False {
                    }
                    frame True {
                      n213 = call "cleanSpool.vi"("error in (no error)"=w434, "Total Img Num"=w435, "strPath"=w432) -> ("error out"=w433:errorcluster)  [unwired: 8 in]
                    }
                  }
                }
                frame #6 {
                  n214 = Wait (ms)(milliseconds to wait=u32 100) -> ()  [unwired: 1 out]
                  n215 = Number To Fractional String(number=w439, precision (6)=1) -> (F-format string=w444:string)  [unwired: 2 in]
                  n216 = Concatenate Strings("movrel z=", w444) -> (w442:string)
                  n217 = call "WriteCmd.vi"("Command"=w442, "VISA resource name"=w441) -> ("error"=w440:errorcluster)  [unwired: 1 in, 1 out]
                  n218 = local write "error out"(w436) -> ()
                }
              }
            }
            n219 = stacked-sequence {
              seq-local: [_ w448 _] -> [_ _ w464]
              tunnel: [_ _ w463] -> w351
              tunnel: w339 -> [_ w452 _]
              tunnel: w338 -> [_ w455 _]
              tunnel: w334 -> [_ w453 _]
              tunnel: "Current Z as Center" -> [_ w450 _]
              tunnel: w328 -> [_ w449 _]
              tunnel: w331 -> [_ _ w462]
              tunnel: w330 -> [_ _ w461]
              frame #0 {
                n220 = local write "EMCCD Status"(FALSE) -> ()
                n221 = local write "Running Status"(0) -> ()
              }
              frame #1 {
                n222 = case shown="True" w450 {
                  tunnel: w452 -> [w459 _]
                  tunnel: [w459 w460] -> w451
                  tunnel: w449 -> [_ w460]
                  frame False {
                  }
                  frame True {
                  }
                }
                n223 = Negate(x=w451) -> (-x=w454:dbl)
                n224 = Number To Fractional String(number=w454, precision (6)=1) -> (F-format string=w457:string)  [unwired: 2 in]
                n225 = Concatenate Strings("movrel z=", w457) -> (w458:string)
                n226 = call "WriteCmd.vi"("error IO"=w453, "Command"=w458, "VISA resource name"=w455) -> ("error"=w448:errorcluster)  [unwired: 1 out]
              }
              frame #2 {
                # "Turn off laser"
                n227 = invoke class="MG17Motor" method="SC_Disable"(reference=w461, error in=w464, "lChanID"=w462) -> (error out=w463:errorcluster)  [unwired: 1 in, 3 out]
              }
            }
          }
        }
      }
      event "Update AcqSetting": Mouse Up {
        n228 = event-data() -> ()  [unwired: 1 in, 8 out]
        n229 = local read "Gain On"() -> (w502:bool)
        n230 = local read "Aquisition Mode"() -> (w513:T2)
        n231 = local read "Accum Num"() -> (w514:u32)
        n232 = To Unsigned Word Integer(number=w513) -> (unsigned 16bit integer=w519:u16)
        n233 = local read "Kinetic Num"() -> (w500:u32)
        n234 = local read "Trigger Mode"() -> (w512:enum16{"Internal", "External"})
        n235 = call <userlib>:"SetAcquisitionMode.vi"("error in (no error)"=w510, "mode"=w519) -> ("error out"=w518:errorcluster)  [unwired: 1 out]
        n236 = To Unsigned Word Integer(number=w512) -> (unsigned 16bit integer=w517:u16)
        n237 = local read "Exposure time (s)"() -> (w511:dbl)
        n238 = call <userlib>:"SetTriggerMode.vi"("error in (no error)"=w518, "mode"=w517) -> ("error out"=w516:errorcluster)  [unwired: 1 out]
        n239 = call <userlib>:"SetExposureTime.vi"("error in (no error)"=w516, "time"=w511) -> ("error out"=w515:errorcluster)  [unwired: 1 out]
        n240 = case shown="\"Kinetics\"" w513 {
          tunnel: w514 -> [_ _ w532 w537]
          tunnel: w515 -> [w528 w529 w531 w536]
          tunnel: [w528 w529 w530 w534] -> w499
          tunnel: w500 -> [_ _ _ w533]
          frame "None", Default {
          }
          frame "Single Scan" {
          }
          frame "Accumulate" {
            n241 = call <userlib>:"SetNumberAccumulations.vi"("error in (no error)"=w531, "number"=w532) -> ("error out"=w530:errorcluster)  [unwired: 1 out]
          }
          frame "Kinetics" {
            n242 = call <userlib>:"SetNumberAccumulations.vi"("error in (no error)"=w536, "number"=w537) -> ("error out"=w535:errorcluster)  [unwired: 1 out]
            n243 = call <userlib>:"SetNumberKinetics.vi"("error in (no error)"=w535, "number"=w533) -> ("error out"=w534:errorcluster)  [unwired: 1 out]
          }
        }
        n244 = case shown="False" w502 {
          tunnel: w499 -> [w521 w527]
          tunnel: [w520 w524] -> w501
          frame False {
            n245 = call <userlib>:"SetEMCCDGain.vi"("error in (no error)"=w521, "gain"=0) -> ("error out"=w520:errorcluster)  [unwired: 1 out]
          }
          frame True {
            # "0-255"
            n246 = call <userlib>:"SetEMGainMode.vi"("error in (no error)"=w527, "mode"=0) -> ("error out"=w525:errorcluster)  [unwired: 1 out]
            n247 = local read "Gain Value"() -> (w523:sgl)
            n248 = call <userlib>:"SetEMCCDGain.vi"("error in (no error)"=w525, "gain"=w523) -> ("error out"=w524:errorcluster)  [unwired: 1 out]
          }
        }
        n249 = call <userlib>:"GetEMCCDGain.vi"("error in (no error)"=w501) -> ("error out"=w504:errorcluster, "gain"=w503:u32)  [unwired: 2 in, 1 out]
        n250 = local write "Get EMCCD Gain"(w503) -> ()
        n251 = call <userlib>:"GetAcquisitionTimings.vi"("error in (no error)"=w504) -> ("exposure"=w509:sgl, "accumulate"=w506:sgl, "kinetic"=w505:sgl, "DLL error code"=w507:u32, "error out"=w508:errorcluster)  [unwired: 10 in]
        n252 = local write "Return from CheckTimings"(w507) -> ()
        n253 = local write "Get Exposure Time"(w509) -> ()
        n254 = local write "Get Kinetic Time"(w505) -> ()
        n255 = local write "Get Accum Time"(w506) -> ()
      }
      event "Update FOV": Value Change {
        n256 = event-data() -> ()  [unwired: 1 in, 6 out]
        n257 = local read "Detector Y Pixels"() -> (w558:i32)
        n258 = local read "Detector X Pixels"() -> (w559:i32)
        n259 = local read "Camera FOV"() -> (w557:T3)
        n260 = case shown="\"Custom FOV\"" w557 {
          tunnel: [w565 w589 w605 w621 w637 w640] -> w553
          tunnel: [w564 w589 w605 w621 w637 w640] -> w554
          tunnel: [w563 w579 w595 w611 w627 w640] -> w555
          tunnel: [w562 w576 w592 w608 w624 w638] -> w556
          tunnel: [w560 w578 w594 w610 w626 w640] -> w552
          tunnel: [w561 w575 w591 w607 w623 w639] -> w551
          tunnel: w559 -> [_ w588 w604 w620 w636 w638]
          tunnel: w558 -> [_ w587 w603 w619 w635 w639]
          tunnel: [w566 w574 w590 w606 w622 w639] -> w549
          tunnel: [w568 w574 w590 w606 w622 w638] -> w550
          frame "Custom FOV" {
            n261 = local read "Xstart"() -> (w563:i32)
            n262 = local read "Xend"() -> (w562:i32)
            n263 = local read "Ystart"() -> (w560:i32)
            n264 = local read "Yend"() -> (w561:i32)
            n265 = Subtract(x=w561, y=w560) -> (x-y=w572:i32)
            n266 = Subtract(x=w562, y=w563) -> (x-y=w573:i32)
            n267 = local read "Xbin"() -> (w565:i32)
            n268 = local read "Ybin"() -> (w564:i32)
            n269 = Increment(x=w572) -> (x+1=w571:i32)
            n270 = Increment(x=w573) -> (x+1=w570:i32)
            n271 = Divide(x=w571, y=w564) -> (x/y=w567:dbl)
            n272 = Divide(x=w570, y=w565) -> (x/y=w569:dbl)
            n273 = To Long Integer(number=w567) -> (32bit integer=w566:i32)
            n274 = To Long Integer(number=w569) -> (32bit integer=w568:i32)
          }
          frame "FOV: 768x768" {
            w574 = 768
            w584 = 2.0
            w589 = 1
            n275 = Subtract(x=w588, y=w574) -> (x-y=w586:i32)
            n276 = Subtract(x=w587, y=w574) -> (x-y=w585:i32)
            n277 = Divide(x=w585, y=w584) -> (x/y=w582:dbl)
            n278 = Divide(x=w586, y=w584) -> (x/y=w583:dbl)
            n279 = Decrement(x=w574) -> (x-1=w577:i32)
            n280 = Round To Nearest(number=w583) -> (nearest integer value=w581:dbl)
            n281 = Round To Nearest(number=w582) -> (nearest integer value=w580:dbl)
            n282 = To Long Integer(number=w581) -> (32bit integer=w579:i32)
            n283 = To Long Integer(number=w580) -> (32bit integer=w578:i32)
            n284 = Add(x=w577, y=w579) -> (x+y=w576:i32)
            n285 = Add(x=w577, y=w578) -> (x+y=w575:i32)
          }
          frame "FOV: 512x512" {
            w590 = 512
            w600 = 2.0
            w605 = 1
            n286 = Subtract(x=w604, y=w590) -> (x-y=w602:i32)
            n287 = Subtract(x=w603, y=w590) -> (x-y=w601:i32)
            n288 = Divide(x=w601, y=w600) -> (x/y=w598:dbl)
            n289 = Divide(x=w602, y=w600) -> (x/y=w599:dbl)
            n290 = Decrement(x=w590) -> (x-1=w593:i32)
            n291 = Round To Nearest(number=w599) -> (nearest integer value=w597:dbl)
            n292 = Round To Nearest(number=w598) -> (nearest integer value=w596:dbl)
            n293 = To Long Integer(number=w597) -> (32bit integer=w595:i32)
            n294 = To Long Integer(number=w596) -> (32bit integer=w594:i32)
            n295 = Add(x=w593, y=w595) -> (x+y=w592:i32)
            n296 = Add(x=w593, y=w594) -> (x+y=w591:i32)
          }
          frame "FOV: 320x320" {
            w606 = 320
            w616 = 2.0
            w621 = 1
            n297 = Subtract(x=w620, y=w606) -> (x-y=w618:i32)
            n298 = Subtract(x=w619, y=w606) -> (x-y=w617:i32)
            n299 = Divide(x=w617, y=w616) -> (x/y=w614:dbl)
            n300 = Divide(x=w618, y=w616) -> (x/y=w615:dbl)
            n301 = Decrement(x=w606) -> (x-1=w609:i32)
            n302 = Round To Nearest(number=w615) -> (nearest integer value=w613:dbl)
            n303 = Round To Nearest(number=w614) -> (nearest integer value=w612:dbl)
            n304 = To Long Integer(number=w613) -> (32bit integer=w611:i32)
            n305 = To Long Integer(number=w612) -> (32bit integer=w610:i32)
            n306 = Add(x=w609, y=w611) -> (x+y=w608:i32)
            n307 = Add(x=w609, y=w610) -> (x+y=w607:i32)
          }
          frame "FOV: 256x256" {
            w622 = 256
            w632 = 2.0
            w637 = 1
            n308 = Subtract(x=w636, y=w622) -> (x-y=w634:i32)
            n309 = Subtract(x=w635, y=w622) -> (x-y=w633:i32)
            n310 = Divide(x=w633, y=w632) -> (x/y=w630:dbl)
            n311 = Divide(x=w634, y=w632) -> (x/y=w631:dbl)
            n312 = Decrement(x=w622) -> (x-1=w625:i32)
            n313 = Round To Nearest(number=w631) -> (nearest integer value=w629:dbl)
            n314 = Round To Nearest(number=w630) -> (nearest integer value=w628:dbl)
            n315 = To Long Integer(number=w629) -> (32bit integer=w627:i32)
            n316 = To Long Integer(number=w628) -> (32bit integer=w626:i32)
            n317 = Add(x=w625, y=w627) -> (x+y=w624:i32)
            n318 = Add(x=w625, y=w626) -> (x+y=w623:i32)
          }
          frame "Full FOV", Default {
            w640 = 1
          }
        }
        n319 = local write "FOV X Pixels"(w550) -> ()
        n320 = local write "FOV Y Pixels"(w549) -> ()
        n321 = call <userlib>:"SetImage.vi"("hbin"=w553, "vbin"=w554, "hstart"=w555, "hend"=w556, "vstart"=w552, "vend"=w551, "error in (no error)"=w548) -> ("error out"=w547:errorcluster)  [unwired: 19 in, 1 out]
        n322 = call <userlib>:"GetAcquisitionTimings.vi"("error in (no error)"=w547) -> ("exposure"=w544:sgl, "accumulate"=w543:sgl, "kinetic"=w542:sgl, "DLL error code"=w541:u32, "error out"=w546:errorcluster)  [unwired: 10 in]
        n323 = call <userlib>:"GetAcquisitionProgress.vi"("error in (no error)"=w546) -> ("error out"=w545:errorcluster, "DLL error code"=w538:u32, "series"=w539:i32, "accum"=w540:i32)  [unwired: 3 in]
        n324 = local write "Get Exposure Time"(w544) -> ()
        n325 = local write "Get Accum Time"(w543) -> ()
        n326 = local write "Get Kinetic Time"(w542) -> ()
        n327 = local write "Return from CheckTimings"(w541) -> ()
        n328 = local write "Return from CheckProcess"(w538) -> ()
        n329 = local write "Get Kinetic Num"(w540) -> ()
        n330 = local write "Get Kinetic Num"(w539) -> ()
      }
      event "Start LIVE": Mouse Up {
        # "Set running mode to Live Preview"
        n331 = event-data() -> ()  [unwired: 1 in, 8 out]
        n332 = flat-sequence {
          tunnel: w643 -> [w645]
          tunnel: [w645] -> w641
          tunnel: w641 -> [w648]
          tunnel: [w646] -> w642
          frame #0 {
            n333 = local write "Running Status"(1) -> ()
          }
          frame #1 {
            w647 = u16 1  # AcquisitionMode
            # "Set Acquisition Mode: Single Scan"
            n334 = call <userlib>:"SetAcquisitionMode.vi"("error in (no error)"=w648, "mode"=w647) -> ("error out"=w646:errorcluster)  [unwired: 1 out]
          }
        }
      }
      event "Stop LIVE": Mouse Up {
        # "Stop Live Preview"
        n335 = event-data() -> ()  [unwired: 1 in, 8 out]
        n336 = flat-sequence {
          tunnel: w652 -> [w654]
          tunnel: [w654] -> w649
          tunnel: [w658] -> w651
          tunnel: w649 -> [w657]
          tunnel: [w660] -> w650
          tunnel: w651 -> [w660]
          frame #0 {
            n337 = local write "Running Status"(0) -> ()
          }
          frame #1 {
            # "Recover Acquisition Mode: As Input"
            n338 = local read "Aquisition Mode"() -> (w656:T2)
            n339 = To Unsigned Word Integer(number=w656) -> (unsigned 16bit integer=w655:u16)
            n340 = call <userlib>:"SetAcquisitionMode.vi"("error in (no error)"=w657, "mode"=w655) -> ("error out"=w658:errorcluster)  [unwired: 1 out]
          }
          frame #2 {
            n341 = local write "EMCCD Status"(FALSE) -> ()
          }
        }
      }
      event "Snap": Mouse Up {
        # "Set to running mode to Data Acquisition"
        n342 = event-data() -> ()  [unwired: 1 in, 8 out]
        n343 = local write "Running Status"(2) -> ()
      }
      event "Acquire": Mouse Up {
        # "Set to running mode to Data Acquisition"
        n344 = event-data() -> ()  [unwired: 1 in, 8 out]
        n345 = local write "Running Status"(3) -> ()
      }
      event "Abort": Mouse Up {
        n346 = event-data() -> ()  [unwired: 1 in, 8 out]
        n347 = local write "Running Status"(0) -> ()
        n348 = call <userlib>:"AbortAcquisition.vi"("error in (no error)"=w666) -> ("error out"=w665:errorcluster)  [unwired: 1 in, 1 out]
      }
      event "Intensity Max": Value Change {
        n349 = event-data() -> ()  [unwired: 1 in, 6 out]
        n350 = property on="Intensity Graph" class="IntGraph (strict)"("ZScale.Maximum"="Intensity Max") -> ()  [unwired: 2 in, 2 out]
      }
      event "Intensity Min": Value Change {
        n351 = event-data() -> ()  [unwired: 1 in, 6 out]
        n352 = property on="Intensity Graph" class="IntGraph (strict)"("ZScale.Minimum"="Intensity Min") -> ()  [unwired: 2 in, 2 out]
      }
      event "Auto Scale": Value Change {
        n353 = event-data() -> ()  [unwired: 1 in, 6 out]
        n354 = property on="Intensity Graph" class="IntGraph (strict)"("ZScale.LooseFit"="Auto Scale") -> ()  [unwired: 2 in, 2 out]
      }
      event "Stage Options": Mouse Up {
        w677 = FALSE
        n355 = event-data() -> ()  [unwired: 1 in, 8 out]
        n356 = call "stage_control.vi"("error in (no error)"=w675, "Close Stage"=w677, "Initialize Stage"=w677, "VISA in"=w676) -> ("error out"=w674:errorcluster)  [unwired: 6 in, 1 out]
      }
      event "Exit": Mouse Up {
        n357 = event-data() -> ()  [unwired: 1 in, 8 out]
      }
      event Panel Close? {
        n358 = event-data() -> ()  [unwired: 1 in, 4 out]
        n359 = event-data("Discard?"=TRUE) -> ()  [unwired: 1 in, 1 out]
      }
    }
    n360 = Wait (ms)(milliseconds to wait=u32 250) -> ()  [unwired: 1 out]
    n361 = local write "error out"(w193) -> ()
  }
  n362 = case shown="False" "Abort" {
    frame False {
    }
    frame True {
    }
  }
  n363 = invoke class="MG17Motor" method="StopCtrl"(reference=w6) -> ()  [unwired: 2 in, 3 out]
  n364 = case shown="False" w1 {
    tunnel: w3 -> [w683 w685]
    tunnel: [w683 w684] -> w2
    frame False {
    }
    frame True {
      # "Turn OFF EMCCD"
      n365 = case shown="True" "TurnOFFCooler" {
        tunnel: w685 -> [w688 w690]
        tunnel: [w688 w689] -> w686
        frame False {
        }
        frame True {
          n366 = stacked-sequence {
            tunnel: w690 -> [w691 w693]
            tunnel: [_ w692] -> w689
            frame #0 {
              n367 = call <userlib>:"CoolerOFF.vi"("error in (no error)"=w691) -> ()  [unwired: 1 in, 2 out]
            }
            frame #1 {
              n368 = while {
                tunnel: w693 -> [_]
                tunnel: [w695] -> w692
                stop <- w697 continue-if-true
                n369 = call <userlib>:"GetTemperature.vi"() -> ("error out"=w695:errorcluster, "temperature"=w694:i32)  [unwired: 4 in, 2 out]
                n370 = local write "Current Temp"(w694) -> ()
                n371 = Wait Until Next ms Multiple(millisecond multiple=u32 500) -> ()  [unwired: 1 out]
                n372 = Less?(x=w694, y=i16 0) -> (x < y?=w697:bool)
              }
            }
          }
        }
      }
      n373 = case shown="Error" w686 {
        tunnel: w686 -> [w700 w701]
        tunnel: [w699 w701] -> w684
        frame No Error {
          n374 = call <userlib>:"ShutDown.vi"("error in (no error)"=w700) -> ("error out"=w699:errorcluster)  [unwired: 1 in, 1 out]
        }
        frame Error {
        }
      }
    }
  }
  n375 = VISA Close(VISA resource name=w13, error in (no error)=w3) -> (error out=w12:errorcluster)
  n376 = Merge Errors(w2, w12) -> (→"error out":errorcluster)
